vi "generate state channels.vi"(11 "tag bus configurable plugin module configuration in":refnum<class "user tag bus module configuration.lvclass">) -> (2 "generated channels":refnum<class "TBM channel.lvclass">[](array[class]), 3 "tag bus configurable plugin module configuration out":refnum<class "user tag bus module configuration.lvclass">)   [LabVIEW 2013, in "user tag bus module configuration.lvclass"]
uses:
  user tag bus module configuration.lvclass
  <vilib>/NI/Tag Bus Module Framework/channel/TBM channel.lvclass
  <vilib>/NI/Tag Bus Module Framework/channel/channel classification.ctl
  <vilib>/NI/Tag Bus/tag/Data Type.ctl
  user tag bus module configuration.lvclass/user tag bus module configuration.ctl
  <vilib>/NI/Tag Bus/tag/tag descriptor.lvclass
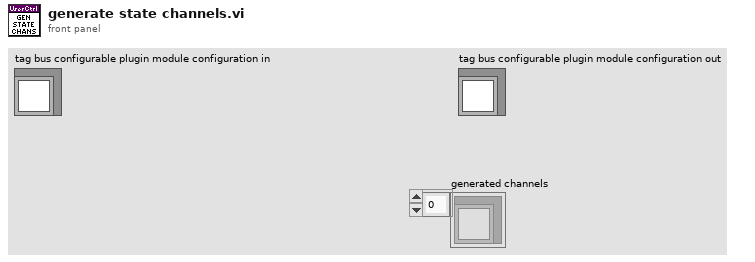
[diagram p1: front panel]
types:
  T1 = typedef "tag bus.lvlib/tag descriptor.lvclass/Data Type.ctl" = enum16{"Double", "Single", "I64", "I32", "I16", "I8", "U64", "U32", "U16", "U8", "Boolean", "String", "Array of Double", "Array of Single", "Array of I64", "Array of I32", "Array of I16", "Array of I8", "Array of U64", "Array of U32", "Array of U16", "Array of U8", "Array of Boolean", "Array of String"}
  T2 = typedef "TBM channel.lvclass/channel classification.ctl" = enum16{"input data", "output data", "processing parameter", "processing result"}
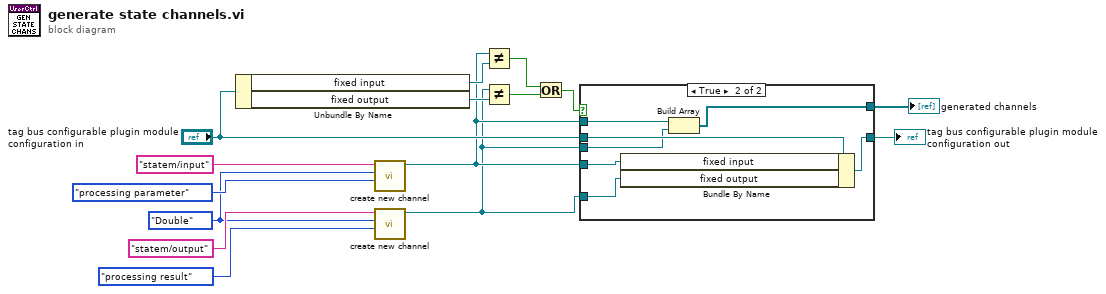
[diagram p0: block diagram]
diagram:
  w10 = Data_Type."Double" ("data type")
  n1 = Unbundle By Name("tag bus configurable plugin module configuration in") -> ("fixed input"=w8:refnum<class "TBM channel.lvclass">, "fixed output"=w7:refnum<class "TBM channel.lvclass">)
  n2 = call <vilib>:"create new channel.vi"("channel classification"=channel_classification."processing parameter", "data type"=w10, "channel name"="statem/input") -> ("channel"=w3:refnum<class "TBM channel.lvclass">)  [unwired: 8 in]
  n3 = call <vilib>:"create new channel.vi"("channel classification"=channel_classification."processing result", "data type"=w10, "channel name"="statem/output") -> ("channel"=w2:refnum<class "TBM channel.lvclass">)  [unwired: 8 in]
  n4 = Not Equal?(x=w3, y=w8) -> (x != y?=w6:bool)
  n5 = Not Equal?(x=w2, y=w7) -> (x != y?=w5:bool)
  n6 = Or(x=w6, y=w5) -> (x .or. y?=w4:bool)
  n7 = case shown="True" w4 {
    tunnel: [w16 w23] -> w15
    tunnel: "tag bus configurable plugin module configuration in" -> [w16 w22]
    tunnel: w3 -> [_ w21]
    tunnel: w2 -> [_ w20]
    tunnel: w3 -> [_ w19]
    tunnel: w2 -> [_ w18]
    tunnel: [_ w17] -> w1
    frame False {
    }
    frame True {
      n8 = Bundle By Name(cluster=w22, "fixed input"=w21, "fixed output"=w20) -> (w23:refnum<class "user tag bus module configuration.lvclass">)
      n9 = Build Array(w19, w18) -> (w17:refnum<class "TBM channel.lvclass">[])
    }
  }
  "tag bus configurable plugin module configuration out" <- w15
  "generated channels" <- w1
